vi "GluePattern_Positioning(SubVI).vi"() -> ()   [LabVIEW 2016]
uses:
  C:/Users/Aerotech/Documents/BNL_ThermomechanicalStave/AerotechLibraries/Bin/Aerotech.A3200.dll
  AerotechLibraries/Bin/Aerotech.A3200.dll
  <vilib>/LabVIEW Interface for Arduino/Type Defs/Arduino Resource.ctl
  <vilib>/LabVIEW Interface for Arduino/Type Defs/Board Type.ctl
  <vilib>/LabVIEW Interface for Arduino/Type Defs/Pin Mode.ctl
  <vilib>/Utility/file.llb/Read Delimited Spreadsheet (DBL).vi
  <vilib>/LabVIEW Interface for Arduino/LabVIEW Interface for Arduino.lvlib
panel:
  out "error out":errorcluster
  out "DX [mm]":dbl
  out "DY [mm]":dbl
  in  "Type of Pattern":u16(ring) items=["Dots", "Lines"]
  out "Arduino Resource":T1={"VISA resource"="COM3", "Board Type"=enum."Uno", "Connection Type"=enum."USB / Serial", "Bytes Per Packet (15)"=15}
  in  "Digital I/O Pin":u8=7
  in  "Final Z":dbl=41.0
  out "Final Position":T3={"Final X"=10.000061631047261, "Final Y"=-16.999877872052817, "Final Z"=35.999801000000005}
  out "Column":i32
  out "Row":i32
  in  "Home?":bool
  out "XYZ Stage Control":refnum<k24>
  in  "File to be processed- Dots":path=path "C:/Users/Aerotech/Documents/BNL_ThermomechanicalStave/1_ModulePlacement/1_GluePatterning/LabVIEW_gluepattern_arraytest.csv"
  in  "Axis Speeds":T4={"vX [mm]"=40.0, "vY [mm]"=40.0, "vZ [mm] "=40.0}
  in  "Go to \ncoordinates":T5={"X [mm]"=10.0, "Y [mm]"=-17.0, "Z [mm] "=36.0}
  in  "Module width [mm]":dbl
  in  "Module length [mm]":dbl
  out "INPUT : Dot":bool[][](array[boolean])=[[TRUE]]
  in  "Duration of glue \ndispensing [s]":dbl=1.5
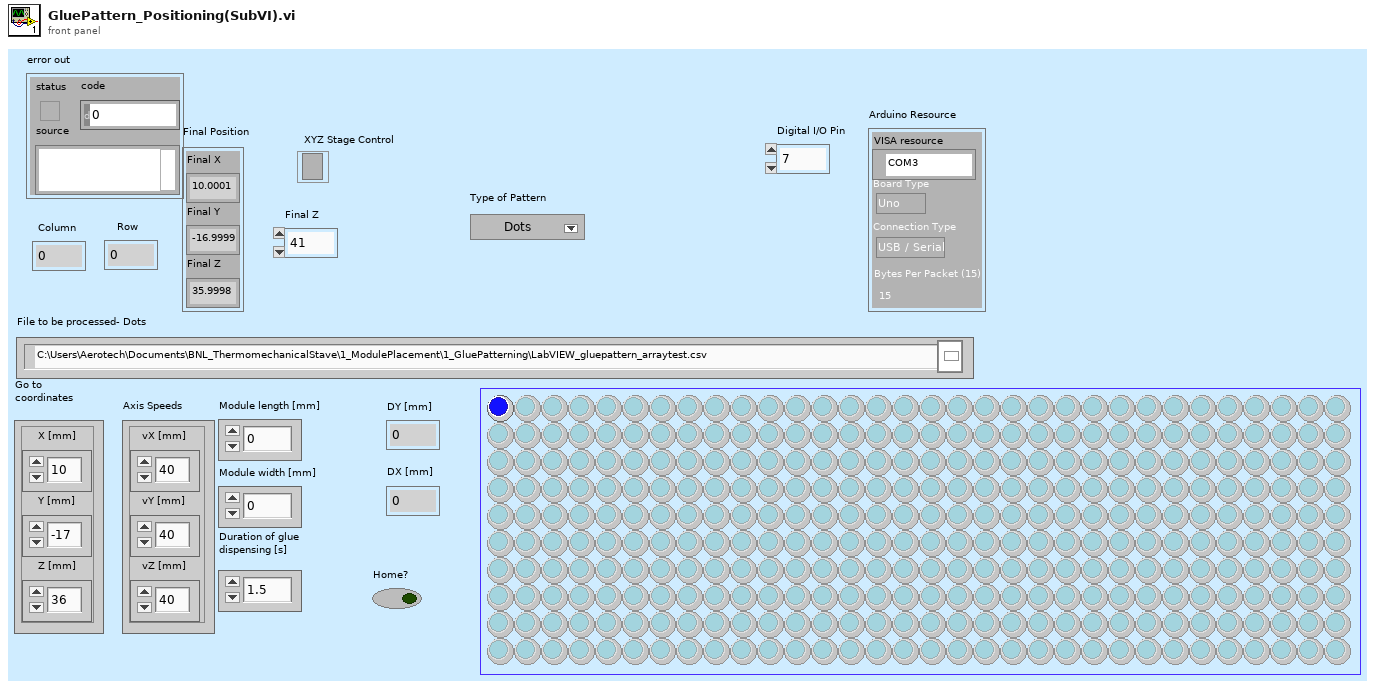
[diagram p1: front panel]
types:
  T1 = typedef "LabVIEW Interface for Arduino.lvlib/Arduino Resource.ctl" = cluster{"VISA resource":refnum<visa-resource-name>, "Board Type":T2, "Connection Type":enum8{"USB / Serial"}, "Bytes Per Packet (15)":u8}
  T2 = typedef "LabVIEW Interface for Arduino.lvlib/Board Type.ctl" = enum16{"Uno", "Dimuelanove w/Atmega 328", "Mega 2560"}
  T3 = cluster{"Final X":dbl, "Final Y":dbl, "Final Z":dbl}
  T4 = cluster{"vX [mm]":dbl, "vY [mm]":dbl, "vZ [mm] ":dbl}
  T5 = cluster{"X [mm]":dbl, "Y [mm]":dbl, "Z [mm] ":dbl}
  T6 = typedef "LabVIEW Interface for Arduino.lvlib/Pin Mode.ctl" = enum8{"Input", "Output"}
  T7 = cluster{"X [mm]":dbl, "Y [mm]":dbl, "Z [mm]":dbl}
  T8 = cluster{"X Position Feedback":dbl, "Y Position Feedback":dbl, "Z Position Feedback":dbl}
  T9 = cluster{"Final X":dbl, "Final Y":dbl, "Z [mm] ":dbl}
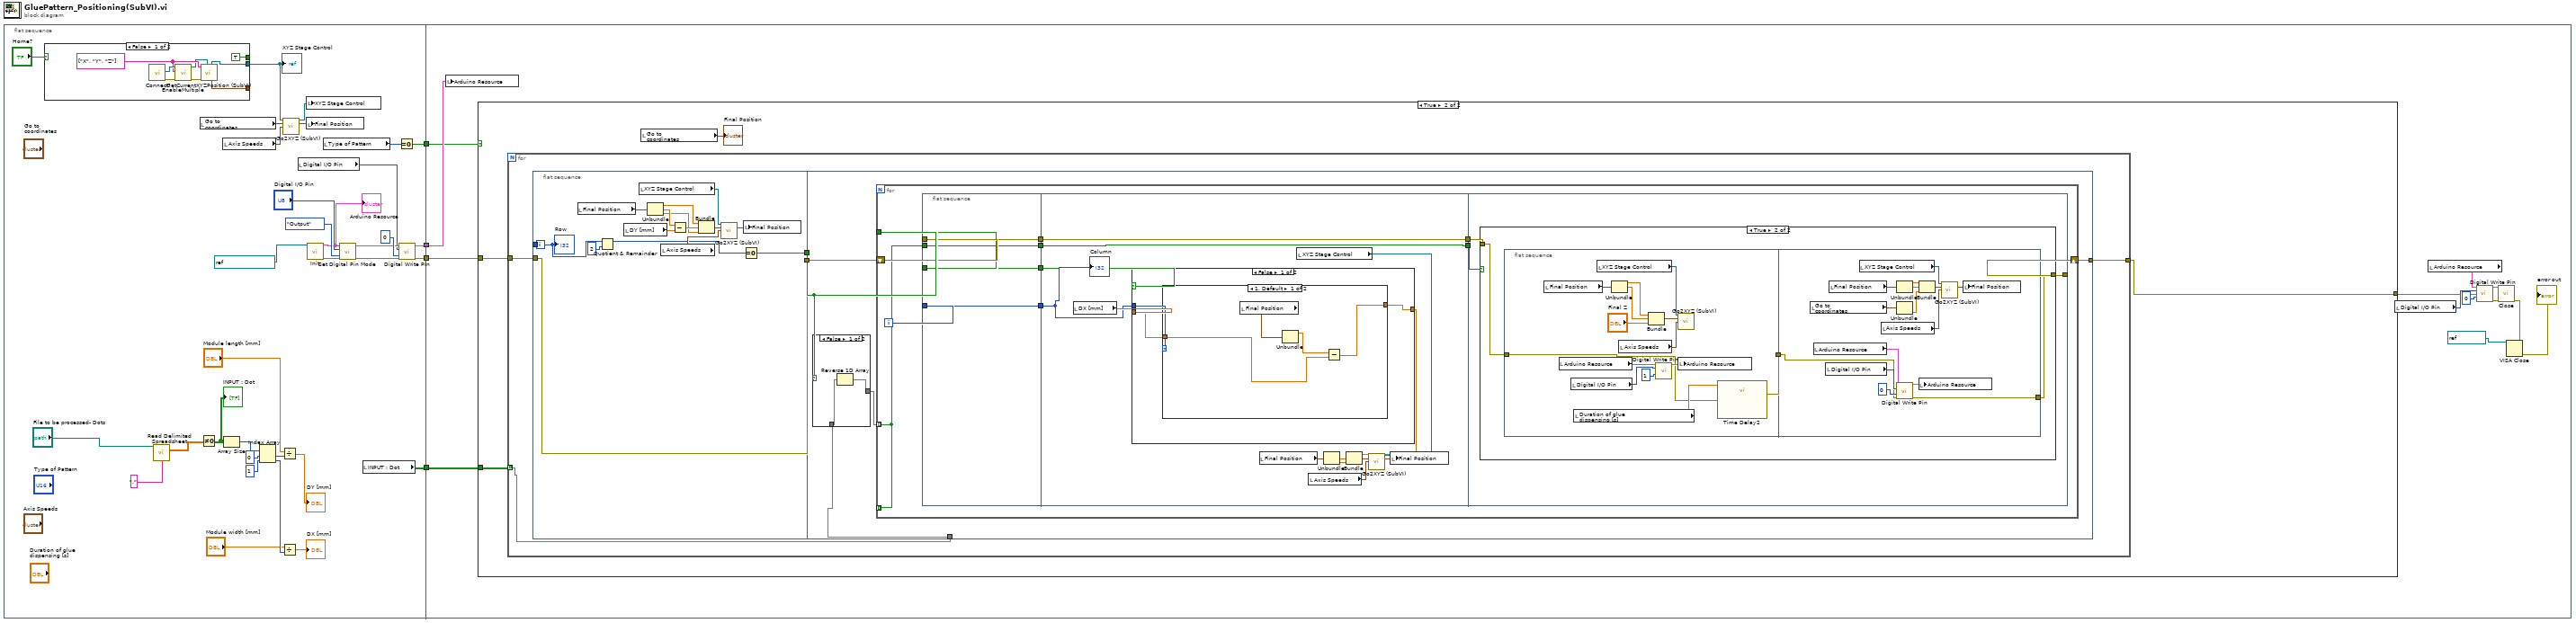
[diagram p0: block diagram]
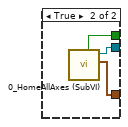
[diagram p2: hidden frame]
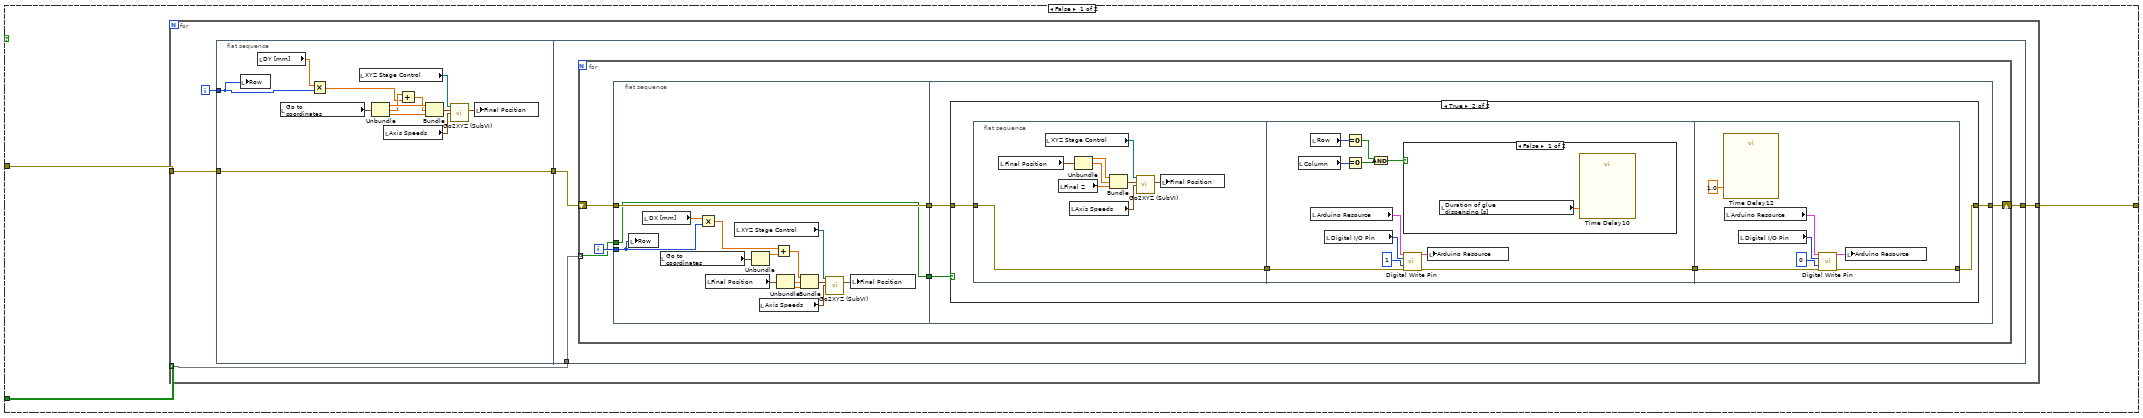
[diagram p3: hidden frame]
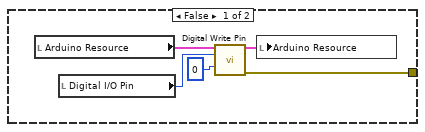
[diagram p4: hidden frame]
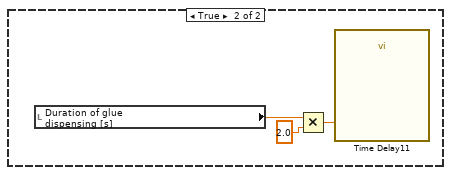
[diagram p5: hidden frame]
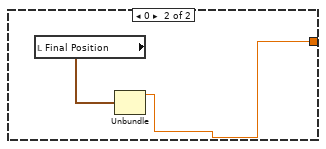
[diagram p7: hidden frame]
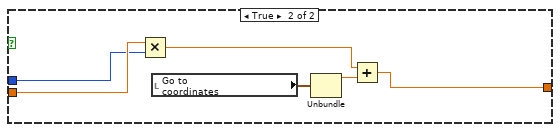
[diagram p8: hidden frame]
diagram:
  n1 = flat-sequence {
    tunnel: [w37] -> w4
    tunnel: [w10] -> w3
    tunnel: [w8] -> w2
    tunnel: [w6] -> w1
    tunnel: w4 -> [w61]
    tunnel: w3 -> [w59]
    tunnel: w2 -> [w60]
    tunnel: w1 -> [w58]
    frame #0 {
      n2 = case shown="False" "Home?" {
        tunnel: [w38 w48] -> _
        tunnel: [TRUE ("completed") w47] -> _
        tunnel: [w40 w46] -> w23
        frame False {
          w42 = string[] ["X", "Y", "Z"] ("Axes Names")
          n3 = call "Connect.vi"() -> ("error out"=w44:errorcluster, "controller"=w43:refnum<k24>)  [unwired: 10 in]
          n4 = call "EnableMultiple.vi"("error in (no error)"=w44, "axis names"=w42, "controller in"=w43) -> ("error out"=w45:errorcluster, "controller out"=w41:refnum<k24>)  [unwired: 7 in]
          n5 = call "GetCurrentXYZPosition (SubVI).vi"(".NET Refnum in - Device"=w41, "error in (no error)"=w45, "Axes Names"=w42) -> ("Current stage position"=w38:T7, ".NET Refnum out  - Device"=w40:refnum<k24>)  [unwired: 3 in, 4 out]
        }
        frame True {
          n6 = call "0_HomeAllAxes (SubVI).vi"() -> ("Homed coordinates"=w48:T8, "controller out"=w46:refnum<k24>, "completed"=w47:bool)  [unwired: 8 in, 1 out]
        }
      }
      "XYZ Stage Control" <- w23
      n7 = call-poly <vilib>:"Read Delimited Spreadsheet.vi"("file path (dialog if empty)"="File to be processed- Dots", "delimiter (\\t)"="," ("delimiter (\\t)")) -> ("all rows"=w35:dbl[][])  [unwired: 8 in, 5 out]
      n8 = local read "Go to \ncoordinates"() -> (w18:T5)
      n9 = Not Equal To 0?(x=w35) -> (x != 0?=w24:bool[][])
      "INPUT : Dot" <- w24
      n10 = local read "Axis Speeds"() -> (w20:T4)
      n11 = Array Size(array=w24) -> (size(s)=w34:i32[])
      n12 = Index Array(array=w34, index #1=0 ("index"), index #2=1 ("index")) -> (element #1=w30:i32, element #2=w29:i32)
      n13 = Divide(x="Module length [mm]", y=w30) -> (x/y=→"DY [mm]":dbl)
      n14 = Divide(x="Module width [mm]", y=w29) -> (x/y=→"DX [mm]":dbl)
      n15 = call "Go2XYZ (SubVI).vi"(".NET Refnum in"=w23, "Go to Coordinates"=w18, "Axis Speeds"=w20) -> (".NET Refnum out"=w19:refnum<k24>, "Final Position"=w21:T3)  [unwired: 8 in, 3 out]
      n16 = local read "Digital I/O Pin"() -> (w9:u8)
      n17 = local write "XYZ Stage Control"(w19) -> ()
      n18 = local write "Final Position"(w21) -> ()
      n19 = call <vilib>:"Init.vi"("VISA resource"=refnum<visa-resource-name> "COM3") -> ("Arduino Resource"=w5:T1, "error out"=w11:errorcluster)  [unwired: 17 in]
      "Arduino Resource" <- w5
      n20 = local read "Type of Pattern"() -> (w7:u16)
      n21 = call <vilib>:"Set Digital Pin Mode.vi"("Arduino Resource"=w5, "Digital I/O Pin"="Digital I/O Pin", "Pin Mode (Input)"=Pin_Mode."Output", "error in"=w11) -> ("Arduino Resource"=w14:T1, "error out"=w15:errorcluster)  [unwired: 10 in]
      n22 = local read "INPUT : Dot"() -> (w8:bool[][])
      n23 = Equal To 0?(x=w7) -> (x = 0?=w6:bool)
      n24 = call <vilib>:"Digital Write Pin.vi"("Arduino Resource"=w14, "Digital I/O Pin (0)"=w9, "Value (0)"=u8 0, "error in"=w15) -> ("Arduino Resource"=w10:T1, "error out"=w37:errorcluster)  [unwired: 10 in]
    }
    frame #1 {
      n25 = local write "Arduino Resource"(w59) -> ()
      n26 = case shown="True" w58 {
        tunnel: w60 -> [w62 w153]
        tunnel: [w63 w152] -> w51
        tunnel: w61 -> [w64 w151]
        frame False {
          n27 = for {
            tunnel: w62 -> [w65] mode=indexing
            tunnel: [w68] -> w63
            tunnel: w64 -> [w66]
            i -> [w69]
            n28 = flat-sequence {
              tunnel: w69 -> [w71]
              tunnel: [w73] -> w67
              tunnel: w66 -> [w73]
              tunnel: w65 -> [w85]
              tunnel: [w84] -> w68
              tunnel: w67 -> [w83]
              frame #0 {
                n29 = local write "Row"(w71) -> ()
                n30 = local read "DY [mm]"() -> (w70:dbl)
                n31 = local read "Go to \ncoordinates"() -> (w79:T5)
                n32 = Multiply(x=w70, y=w71) -> (x*y=w75:dbl)
                n33 = local read "XYZ Stage Control"() -> (w81:refnum<k24>)
                n34 = Unbundle(w79) -> ("X [mm]"=w78:dbl, "Y [mm]"=w76:dbl, "Z [mm]"=w77:dbl)
                n35 = local read "Axis Speeds"() -> (w82:T4)
                n36 = Add(x=w76, y=w75) -> (x+y=w74:dbl)
                n37 = Bundle("X [mm]"=w78, w74, "Z [mm]"=w77) -> (w80:cluster{"X [mm]":dbl, dbl, "Z [mm] ":dbl})  [unwired: 1 in]
                n38 = call "Go2XYZ (SubVI).vi"(".NET Refnum in"=w81, "Go to Coordinates"=w80, "Axis Speeds"=w82) -> ("Final Position"=w72:T3)  [unwired: 8 in, 4 out]
                n39 = local write "Final Position"(w72) -> ()
              }
              frame #1 {
                n40 = for {
                  shift-right: [w86] -> w84
                  shift-left: w83 -> [w90]
                  tunnel: w85 -> [w87] mode=indexing
                  i -> [w91]
                  n41 = flat-sequence {
                    tunnel: w91 -> [w94]
                    tunnel: w90 -> [w104]
                    tunnel: [w104] -> w89
                    tunnel: [w103] -> w88
                    tunnel: w87 -> [w103]
                    tunnel: w89 -> [w109]
                    tunnel: w88 -> [w107]
                    tunnel: [w108] -> w86
                    frame #0 {
                      n42 = local write "Row"(w94) -> ()
                      n43 = local read "DX [mm]"() -> (w92:dbl)
                      n44 = local read "Go to \ncoordinates"() -> (w98:T5)
                      n45 = Multiply(x=w92, y=w94) -> (x*y=w97:dbl)
                      n46 = local read "Final Position"() -> (w93:T3)
                      n47 = local read "XYZ Stage Control"() -> (w105:refnum<k24>)
                      n48 = Unbundle(w98) -> ("X [mm]"=w96:dbl)  [unwired: 2 out]
                      n49 = local read "Axis Speeds"() -> (w106:T4)
                      n50 = Add(x=w97, y=w96) -> (x+y=w95:dbl)
                      n51 = Unbundle(w93) -> ("Final Y"=w102:dbl, "Final Z"=w99:dbl)  [unwired: 1 out]
                      n52 = Bundle(w95, "Final Y"=w102, "Final Z"=w99) -> (w100:cluster{dbl, "Final Y":dbl, "Final Z":dbl})  [unwired: 1 in]
                      n53 = call "Go2XYZ (SubVI).vi"(".NET Refnum in"=w105, "Go to Coordinates"=w100, "Axis Speeds"=w106) -> ("Final Position"=w101:T3)  [unwired: 8 in, 4 out]
                      n54 = local write "Final Position"(w101) -> ()
                    }
                    frame #1 {
                      n55 = case shown="True" w107 {
                        tunnel: [w113 w116] -> w108
                        tunnel: w109 -> [_ w117]
                        frame False {
                          n56 = local read "Arduino Resource"() -> (w112:T1)
                          n57 = local read "Digital I/O Pin"() -> (w111:u8)
                          n58 = call <vilib>:"Digital Write Pin.vi"("Arduino Resource"=w112, "Digital I/O Pin (0)"=w111, "Value (0)"=u8 0) -> ("Arduino Resource"=w110:T1, "error out"=w113:errorcluster)  [unwired: 11 in]
                          n59 = local write "Arduino Resource"(w110) -> ()
                        }
                        frame True {
                          n60 = flat-sequence {
                            tunnel: [w125] -> w118
                            tunnel: w117 -> [w125]
                            tunnel: w118 -> [w133]
                            tunnel: [w137] -> w115
                            tunnel: [w143] -> w116
                            tunnel: w115 -> [w144]
                            frame #0 {
                              n61 = local read "Final Position"() -> (w123:T3)
                              n62 = local read "XYZ Stage Control"() -> (w126:refnum<k24>)
                              n63 = local read "Final Z"() -> (w120:dbl)
                              n64 = local read "Axis Speeds"() -> (w127:T4)
                              n65 = Unbundle(w123) -> ("Final X"=w122:dbl, "Final Y"=w121:dbl)  [unwired: 1 out]
                              n66 = Bundle("Final X"=w122, "Final Y"=w121, "Final Z"=w120) -> (w124:T3)  [unwired: 1 in]
                              n67 = call "Go2XYZ (SubVI).vi"(".NET Refnum in"=w126, "Go to Coordinates"=w124, "Axis Speeds"=w127) -> ("Final Position"=w119:T3)  [unwired: 8 in, 4 out]
                              n68 = local write "Final Position"(w119) -> ()
                            }
                            frame #1 {
                              n69 = local read "Column"() -> (w130:i32)
                              n70 = local read "Row"() -> (w132:i32)
                              n71 = local read "Arduino Resource"() -> (w136:T1)
                              n72 = local read "Digital I/O Pin"() -> (w135:u8)
                              n73 = Equal To 0?(x=w132) -> (x = 0?=w131:bool)
                              n74 = Equal To 0?(x=w130) -> (x = 0?=w129:bool)
                              n75 = And(x=w131, y=w129) -> (x .and. y?=w128:bool)
                              n76 = case shown="False" w128 {
                                frame False {
                                n77 = local read "Duration of glue \ndispensing [s]"() -> (w139:dbl)
                                n78 = call "Time Delay10"("Delay Time (s)"=w139) -> ()  [unwired: 10 in, 1 out]
                                }
                                frame True {
                                n79 = local read "Duration of glue \ndispensing [s]"() -> (w141:dbl)
                                n80 = Multiply(x=w141, y=2.0) -> (x*y=w140:dbl)
                                n81 = call "Time Delay11"("Delay Time (s)"=w140) -> ()  [unwired: 10 in, 1 out]
                                }
                              }
                              n82 = call <vilib>:"Digital Write Pin.vi"("Arduino Resource"=w136, "Digital I/O Pin (0)"=w135, "Value (0)"=u8 1, "error in"=w133) -> ("Arduino Resource"=w134:T1, "error out"=w137:errorcluster)  [unwired: 10 in]
                              n83 = local write "Arduino Resource"(w134) -> ()
                            }
                            frame #2 {
                              n84 = call "Time Delay12"("Delay Time (s)"=1.0) -> ()  [unwired: 10 in, 1 out]
                              n85 = local read "Arduino Resource"() -> (w145:T1)
                              n86 = local read "Digital I/O Pin"() -> (w146:u8)
                              n87 = call <vilib>:"Digital Write Pin.vi"("Arduino Resource"=w145, "Digital I/O Pin (0)"=w146, "Value (0)"=u8 0, "error in"=w144) -> ("Arduino Resource"=w148:T1, "error out"=w143:errorcluster)  [unwired: 10 in]
                              n88 = local write "Arduino Resource"(w148) -> ()
                            }
                          }
                        }
                      }
                    }
                  }
                }
              }
            }
          }
        }
        frame True {
          n89 = for {
            tunnel: w153 -> [w154] mode=indexing
            tunnel: [w158] -> w152
            tunnel: w151 -> [w156]
            i -> [w159]
            n90 = flat-sequence {
              tunnel: w159 -> [w163]
              tunnel: [w174] -> w157
              tunnel: w156 -> [w174]
              tunnel: [w160] -> w155
              tunnel: w154 -> [w177]
              tunnel: [w179] -> w158
              tunnel: w157 -> [w178]
              tunnel: w155 -> [w175]
              frame #0 {
                n91 = local read "Final Position"() -> (w168:T3)
                n92 = Quotient & Remainder(x=w163, y=2) -> (x-y*floor(x/y)=w161:i32)  [unwired: 1 out]
                n93 = local read "DY [mm]"() -> (w164:dbl)
                n94 = local read "XYZ Stage Control"() -> (w166:refnum<k24>)
                n95 = Unbundle(w168) -> ("Final X"=w169:dbl, "Final Y"=w171:dbl, "Final Z"=w170:dbl)
                n96 = local read "Axis Speeds"() -> (w173:T4)
                n97 = Subtract(x=w171, y=w164) -> (x-y=w172:dbl)
                n98 = Bundle("Final X"=w169, w172, "Final Z"=w170) -> (w167:cluster{"Final X":dbl, dbl, "Final Z":dbl})  [unwired: 1 in]
                n99 = call "Go2XYZ (SubVI).vi"(".NET Refnum in"=w166, "Go to Coordinates"=w167, "Axis Speeds"=w173) -> ("Final Position"=w165:T3)  [unwired: 8 in, 4 out]
                n100 = Equal To 0?(x=w161) -> (x = 0?=w160:bool)
                n101 = local write "Final Position"(w165) -> ()
                "Row" <- w163
              }
              frame #1 {
                n102 = case shown="False" w175 {
                  tunnel: w177 -> [w181 w182]
                  tunnel: [w180 w182] -> w176
                  frame False {
                    n103 = Reverse 1D Array(array=w181) -> (reversed array=w180:bool[])
                  }
                  frame True {
                  }
                }
                n104 = for {
                  shift-right: [w189] -> w179
                  shift-left: w178 -> [w192]
                  tunnel: [w183] -> _ mode=indexing
                  tunnel: w175 -> [w188]
                  tunnel: w176 -> [w183] mode=indexing
                  i -> [w193]
                  n105 = flat-sequence {
                    tunnel: w188 -> [w194]
                    tunnel: w183 -> [w195]
                    tunnel: w192 -> [w196]
                    tunnel: w193 -> [w197]
                    tunnel: [w197] -> w187
                    tunnel: [w196] -> w186
                    tunnel: [w195] -> w185
                    tunnel: [w194] -> w184
                    tunnel: [w206] -> w191
                    tunnel: [w198] -> w190
                    tunnel: w187 -> [w207]
                    tunnel: w186 -> [w206]
                    tunnel: w185 -> [w198]
                    tunnel: w184 -> [w199]
                    tunnel: w191 -> [w228]
                    tunnel: w190 -> [w226]
                    tunnel: [w227] -> w189
                    frame #0 {
                    }
                    frame #1 {
                      n106 = local read "DX [mm]"() -> (w208:dbl)
                      n107 = case shown="False" w199 {
                        tunnel: w208 -> [w212 w225]
                        tunnel: w207 -> [w211 w220]
                        tunnel: [w213 w221] -> w200
                        frame False {
                          n108 = case shown="1, Default" w211 {
                            tunnel: [w217 w218] -> w213
                            tunnel: w212 -> [w216 _]
                            frame 1, Default {
                              n109 = local read "Final Position"() -> (w215:T3)
                              n110 = Unbundle(w215) -> ("Final X"=w214:dbl)  [unwired: 2 out]
                              n111 = Subtract(x=w214, y=w216) -> (x-y=w217:dbl)
                            }
                            frame 0 {
                              n112 = local read "Final Position"() -> (w219:T3)
                              n113 = Unbundle(w219) -> ("Final X"=w218:dbl)  [unwired: 2 out]
                            }
                          }
                        }
                        frame True {
                          n114 = Multiply(x=w225, y=w220) -> (x*y=w223:dbl)
                          n115 = local read "Go to \ncoordinates"() -> (w224:T5)
                          n116 = Unbundle(w224) -> ("X [mm]"=w222:dbl)  [unwired: 2 out]
                          n117 = Add(x=w223, y=w222) -> (x+y=w221:dbl)
                        }
                      }
                      n118 = local read "Final Position"() -> (w205:T3)
                      n119 = local read "XYZ Stage Control"() -> (w209:refnum<k24>)
                      n120 = local read "Axis Speeds"() -> (w210:T4)
                      n121 = Unbundle(w205) -> ("Final Y"=w204:dbl, "Final Z"=w201:dbl)  [unwired: 1 out]
                      n122 = Bundle("Final X"=w200, "Final Y"=w204, "Final Z"=w201) -> (w202:T3)  [unwired: 1 in]
                      n123 = call "Go2XYZ (SubVI).vi"(".NET Refnum in"=w209, "Go to Coordinates"=w202, "Axis Speeds"=w210) -> ("Final Position"=w203:T3)  [unwired: 8 in, 4 out]
                      n124 = local write "Final Position"(w203) -> ()
                      "Column" <- w207
                    }
                    frame #2 {
                      n125 = case shown="True" w226 {
                        tunnel: [w229 w231] -> w227
                        tunnel: w228 -> [w229 w232]
                        frame False {
                        }
                        frame True {
                          n126 = flat-sequence {
                            tunnel: [w233] -> w230
                            tunnel: w232 -> [w234]
                            tunnel: [w256] -> w231
                            tunnel: w230 -> [w257]
                            frame #0 {
                              n127 = local read "Final Position"() -> (w242:T3)
                              n128 = local read "Arduino Resource"() -> (w237:T1)
                              n129 = local read "Digital I/O Pin"() -> (w238:u8)
                              n130 = local read "Duration of glue \ndispensing [s]"() -> (w235:dbl)
                              n131 = local read "XYZ Stage Control"() -> (w244:refnum<k24>)
                              n132 = Unbundle(w242) -> ("Final X"=w241:dbl, "Final Y"=w240:dbl)  [unwired: 1 out]
                              n133 = local read "Axis Speeds"() -> (w245:T4)
                              n134 = Bundle("Final X"=w241, "Final Y"=w240, "Final Z"="Final Z") -> (w243:T3)  [unwired: 1 in]
                              n135 = call <vilib>:"Digital Write Pin.vi"("Arduino Resource"=w237, "Digital I/O Pin (0)"=w238, "Value (0)"=u8 1) -> ("Arduino Resource"=w239:T1)  [unwired: 11 in, 1 out]
                              n136 = call "Go2XYZ (SubVI).vi"(".NET Refnum in"=w244, "Go to Coordinates"=w243, "Axis Speeds"=w245) -> ()  [unwired: 8 in, 5 out]
                              n137 = local write "Arduino Resource"(w239) -> ()
                              n138 = call "Time Delay2"("error in (no error)"=w234, "Delay Time (s)"=w235) -> ("error out"=w233:errorcluster)  [unwired: 9 in]
                            }
                            frame #1 {
                              n139 = local read "Go to \ncoordinates"() -> (w254:T5)
                              n140 = local read "Arduino Resource"() -> (w258:T1)
                              n141 = local read "Digital I/O Pin"() -> (w259:u8)
                              n142 = local read "Final Position"() -> (w255:T3)
                              n143 = local read "XYZ Stage Control"() -> (w248:refnum<k24>)
                              n144 = local read "Axis Speeds"() -> (w249:T4)
                              n145 = Unbundle(w255) -> ("Final X"=w253:dbl, "Final Y"=w252:dbl)  [unwired: 1 out]
                              n146 = Unbundle(w254) -> ("Z [mm]"=w251:dbl)  [unwired: 2 out]
                              n147 = call <vilib>:"Digital Write Pin.vi"("Arduino Resource"=w258, "Digital I/O Pin (0)"=w259, "Value (0)"=u8 0, "error in"=w257) -> ("Arduino Resource"=w261:T1, "error out"=w256:errorcluster)  [unwired: 10 in]
                              n148 = Bundle("Final X"=w253, "Final Y"=w252, "Z [mm]"=w251) -> (w250:T9)  [unwired: 1 in]
                              n149 = local write "Arduino Resource"(w261) -> ()
                              n150 = call "Go2XYZ (SubVI).vi"(".NET Refnum in"=w248, "Go to Coordinates"=w250, "Axis Speeds"=w249) -> ("Final Position"=w247:T3)  [unwired: 8 in, 4 out]
                              n151 = local write "Final Position"(w247) -> ()
                            }
                          }
                        }
                      }
                    }
                  }
                }
              }
            }
          }
          n152 = local read "Go to \ncoordinates"() -> (→"Final Position":T5)
        }
      }
      n153 = local read "Digital I/O Pin"() -> (w56:u8)
      n154 = local read "Arduino Resource"() -> (w55:T1)
      n155 = call <vilib>:"Digital Write Pin.vi"("Arduino Resource"=w55, "Digital I/O Pin (0)"=w56, "Value (0)"=u8 0, "error in"=w51) -> ("Arduino Resource"=w53:T1, "error out"=w52:errorcluster)  [unwired: 10 in]
      n156 = call <vilib>:"Close.vi"("Arduino Resource"=w53, "error in"=w52) -> ("error out"=w50:errorcluster)  [unwired: 13 in]
      n157 = VISA Close(VISA resource name=refnum<visa-resource-name> "COM3", error in (no error)=w50) -> (error out=→"error out":errorcluster)
    }
  }
